vi "InitERAConfig.vi"(7 "Ring Refnum":refnum<vi>, 8 "error in (no error)":errorcluster, 10 "ERA Configuration":T1={"Threshold"=3.0, "Model Order"=1, "Preprocessing "={"order"=0, "f_lo"=0.0, "f_hi"=0.0, "R_down"=0}}, 11 "RingdownPlugin":refnum<class "EraPlugin.lvclass">=refnum) -> (0 "error out":errorcluster, 2 "ERA Configuration":T1, 3 "RingdownPlugin":refnum<class "EraPlugin.lvclass">)   [LabVIEW 2017, in "AppPlugins.lvlib" / "ERAPlugin.lvclass"]
uses:
  EraPlugin.lvclass
  ERAConfig.ctl
  Mode Estimation/COM_Preproc Parameters.ctl
  PublicAPI/TypeDef/ePhase.ctl
  EraPlugin.lvclass/EraPlugin.ctl
  <vilib>/Utility/miscctls.llb/LVStringsAndValuesArrayTypeDef_U16.ctl
  Accessors/Read RingdownConfig.vi
  <vilib>/Utility/error.llb/Error Cluster From Error Code.vi
  <vilib>/ErrorRing/Error Ring.xnode
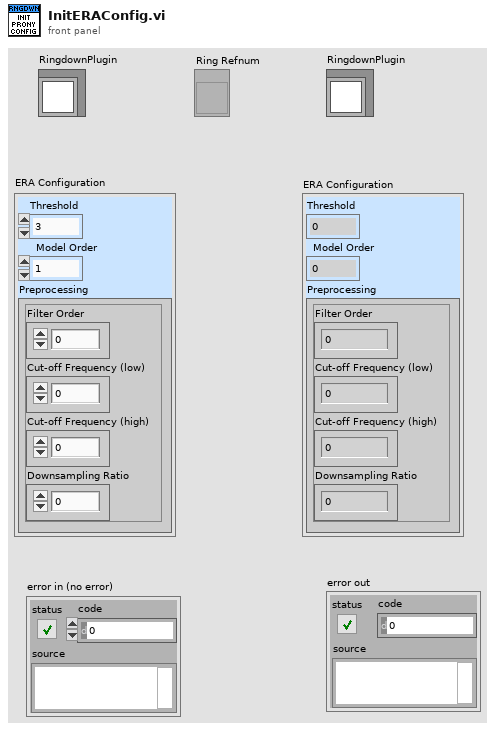
[diagram p1: front panel]
types:
  T1 = typedef "AppPlugins.lvlib/ERAPlugin.lvclass/ERAConfig.ctl" = cluster{"Threshold":dbl, "Model Order":i32, "Preprocessing ":T2}
  T2 = typedef "AppPlugins.lvlib/EraPlugin.lvclass/COM_Preproc Parameters.ctl" = cluster{"order":i32, "f_lo":dbl, "f_hi":dbl, "R_down":i32}
  T3 = typedef "AppPlugins.lvlib/ERAPlugin.lvclass/RingdownConfig.ctl" = cluster{"Config":cluster{"p_SysOdr":i32, "dThres":dbl, "Preproc":cluster{"order":i32, "f_lo":dbl, "f_hi":dbl, "R_down":i32}}, "V index":i32, "I index":i32, "PosSeq":bool}
  T4 = cluster{"p_SysOdr":i32, "dThres":dbl, "Preproc":cluster{"order":i32, "f_lo":dbl, "f_hi":dbl, "R_down":i32}}
  T5 = typedef "AppPlugins.lvlib/ERAPlugin.lvclass/ePhase.ctl" = u16
  T6 = typedef "LVStringsAndValuesArrayTypeDef_U16.ctl" = cluster{"String":string, "Value":u16}[]
  T7 = typedef "ePhase.ctl" = u16
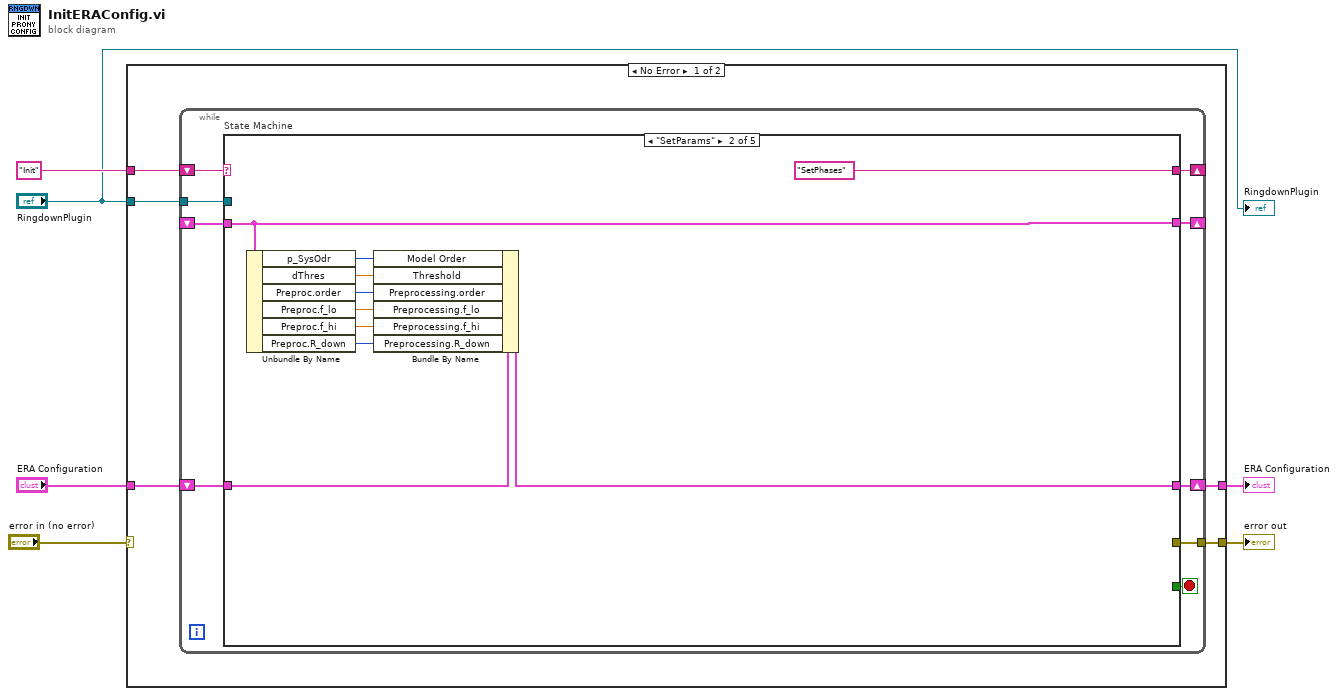
[diagram p0: block diagram]
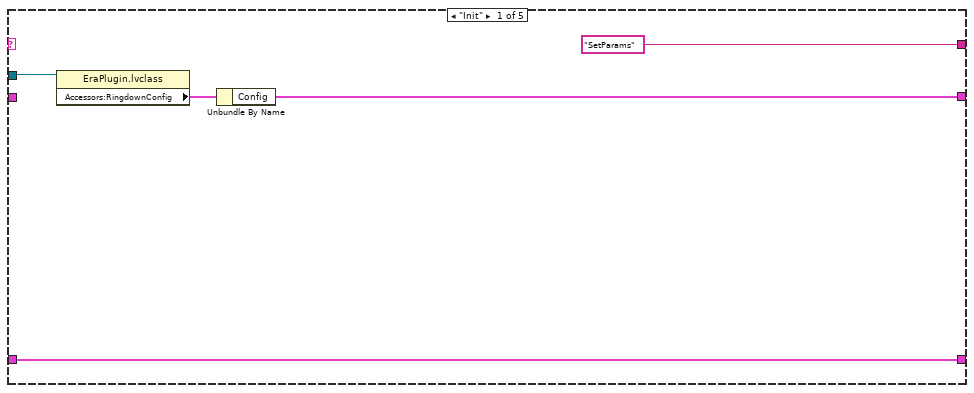
[diagram p2: hidden frame]
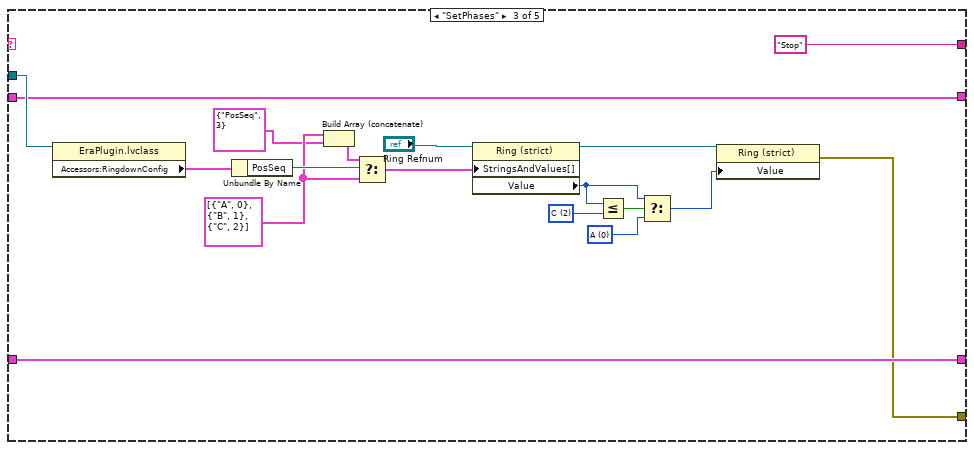
[diagram p3: hidden frame]
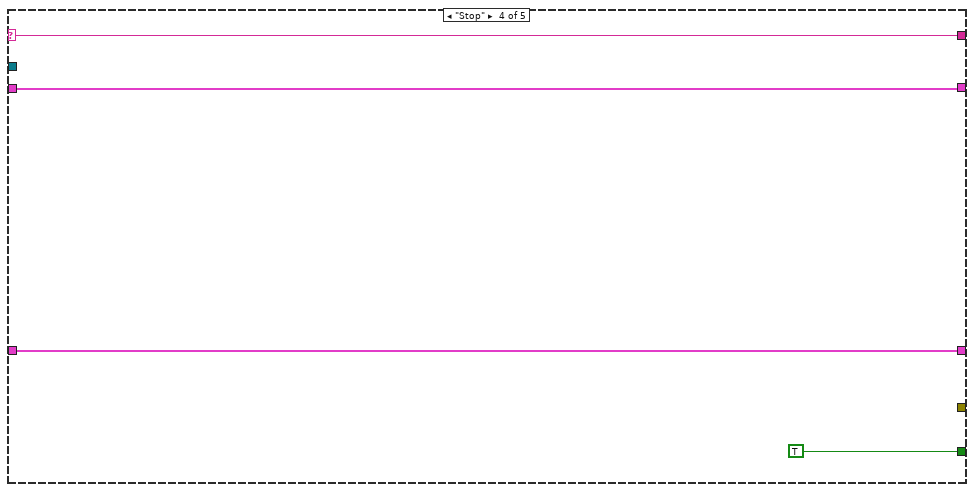
[diagram p4: hidden frame]
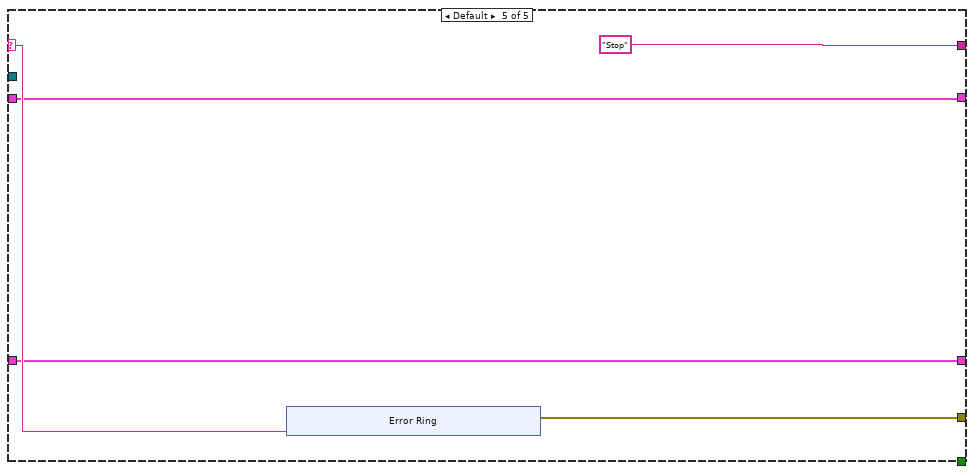
[diagram p5: hidden frame]
diagram:
  n1 = case shown="No Error" "error in (no error)" {
    selector: "error in (no error)" -> [_ w71]
    tunnel: "Init" -> [w11 _]
    tunnel: "ERA Configuration" -> [w10 w70]
    tunnel: "RingdownPlugin" -> [w9 _]
    tunnel: [w8 w70] -> w3
    tunnel: [w7 w71] -> w2
    frame No Error {
      n2 = while {
        shift-right: [w16] -> _
        shift-left: w11 -> [w20]
        shift-right: [w17] -> _
        shift-left: _ -> [w19]
        tunnel: w9 -> [w18]
        shift-right: [w14] -> w8
        shift-left: w10 -> [w15]
        tunnel: [w12] -> w7
        stop <- w13 stop-if-true
        n3 = case "State Machine" shown="\"SetParams\"" w20 {
          selector: w20 -> [_ _ _ w56 w61]
          tunnel: w19 -> [_ w30 w49 w55 w60]
          tunnel: w18 -> [w24 _ w53 _ _]
          tunnel: [w21 w30 w49 w55 w60] -> w17
          tunnel: ["SetParams" "SetPhases" "Stop" w56 "Stop"] -> w16
          tunnel: w15 -> [w22 w35 w47 w54 w59]
          tunnel: [w22 w34 w47 w54 w59] -> w14
          tunnel: [_ _ _ TRUE _] -> w13
          tunnel: [_ _ w40 _ w58] -> w12
          frame "Init" {
            n4 = property class="EraPlugin.lvclass"(reference=w24) -> ("Accessors:RingdownConfig"=w25:T3)  [unwired: 1 in, 2 out]
            n5 = Unbundle By Name(w25) -> ("Config"=w21:T4)
          }
          frame "SetParams" {
            n6 = Unbundle By Name(w30) -> ("p_SysOdr"=w33:i32, "dThres"=w32:dbl, "Preproc.order"=w29:i32, "Preproc.f_lo"=w28:dbl, "Preproc.f_hi"=w27:dbl, "Preproc.R_down"=w26:i32)
            n7 = Bundle By Name(cluster=w35, "Model Order"=w33, "Threshold"=w32, "Preprocessing.order"=w29, "Preprocessing.f_lo"=w28, "Preprocessing.f_hi"=w27, "Preprocessing.R_down"=w26) -> (w34:T1)
          }
          frame "SetPhases" {
            w36 = T5 0 items=["A", "B", "C", "PosSeq"] ("y")
            w42 = T5 2 items=["A", "B", "C", "PosSeq"] ("y")
            w46 = T6 [{"String"="A", "Value"=0}, {"String"="B", "Value"=1}, {"String"="C", "Value"=2}] ("Strings And Values []")
            n8 = property class="EraPlugin.lvclass"(reference=w53) -> ("Accessors:RingdownConfig"=w52:T3)  [unwired: 1 in, 2 out]
            n9 = Unbundle By Name(w52) -> ("PosSeq"=w51:bool)
            n10 = Build Array (concatenate)(w46, cluster{"String":string, "Value":i32} {"String"="PosSeq", "Value"=3}) -> (w50:cluster{"String":string, "Value":i32}[])
            n11 = Select(t=w50, s=w51, f=w46) -> (s? t:f=w44:cluster{"String":string, "Value":i32}[])
            n12 = property class="Ring (strict)"(reference="Ring Refnum", "StringsAndValues[]"=w44) -> (reference out=w41:refnum<vi>, "Value"=w38:T7)  [unwired: 1 in, 1 out]
            n13 = Less Or Equal?(x=w38, y=w42) -> (x <= y?=w37:bool)
            n14 = Select(t=w38, s=w37, f=w36) -> (s? t:f=w39:T5)
            n15 = property class="Ring (strict)"(reference=w41, "Value"=w39) -> (error out=w40:errorcluster)  [unwired: 1 in, 1 out]
          }
          frame "Stop" {
          }
          frame Default {
            n16 = xnode "Error Ring"("parameter 0"=w61) -> ("error out"=w58:errorcluster)
          }
        }
      }
    }
    frame Error {
    }
  }
  "ERA Configuration" <- w3
  "error out" <- w2
  "RingdownPlugin" <- "RingdownPlugin"
